vi "Read pointer.vi"(11 "connection creator in":refnum<class "connection creator.lvclass">) -> (2 "pointer":refnum<data-value>)   [LabVIEW 2016, in "connection creator.lvclass"]
uses:
  connection creator.lvclass
  connection creator.lvclass/connection creator.ctl
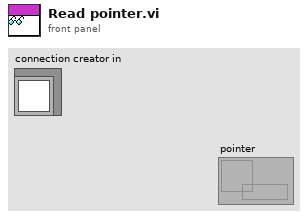
[diagram p1: front panel]
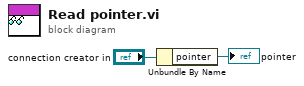
[diagram p0: block diagram]
diagram:
  n1 = Unbundle By Name("connection creator in") -> ("pointer"=→"pointer":refnum<data-value>)
